vi "Verify Cancel.vi"(8 "error in":errorcluster) -> (0 "error out":errorcluster)   [LabVIEW 2021]
uses:
  <resource>/plugins/NIIconEditor/Controls/Undo Redo Action.ctl
panel:
  out "curr pointer":i32
  out "String":string
  out "Preview Empty String?":bool
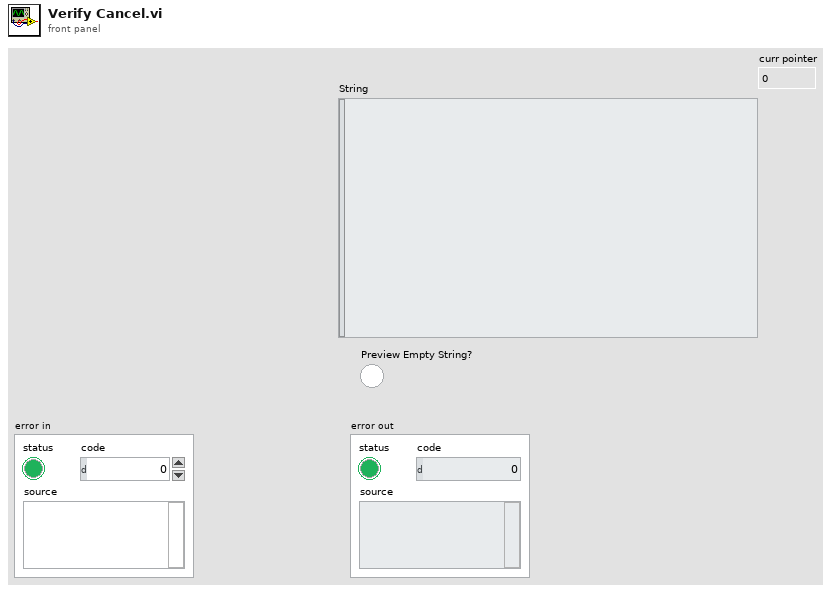
[diagram p1: front panel]
types:
  T1 = typedef "Undo Redo Action.ctl" = enum16{"Init", "Add", "Redo", "Undo", "Undo Preview"}
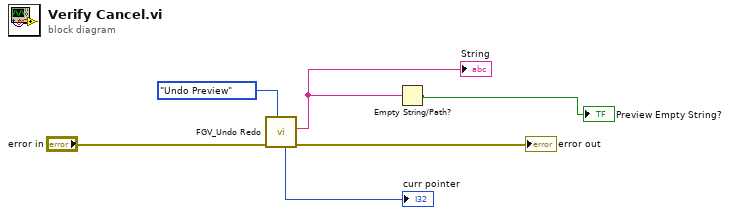
[diagram p0: block diagram]
diagram:
  n1 = call <resource>:"FGV_Undo Redo.vi"("Action"=Undo_Redo_Action."Undo Preview", "error in (no error)"="error in") -> ("error out"=→"error out":errorcluster, "Data out"=w2:string, "curr pointer"=→"curr pointer":i32)  [unwired: 6 in, 1 out]
  "String" <- w2
  n2 = Empty String/Path?(string/path=w2) -> (empty?=→"Preview Empty String?":bool)
